vi "waitForRisEdge.vi"(3 "delay(ticks)":u32, 4 "MCSSelectTrigger":T1) -> (1 "out":bool, 2 "triggered?":bool)   [LabVIEW 2014]
uses:
  Controls/selectTrigger.ctl
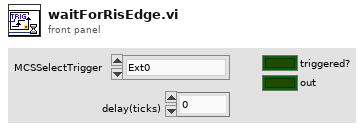
[diagram p1: front panel]
types:
  T1 = typedef "selectTrigger.ctl" = enum8{"Ext0", "Ext1", "Ext2", "Ext3", "Ext4", "Ext5", "Ext6", "Ext7", "Int0", "Int1", "Int2", "Int3", "Int4", "Int5", "Int6", "Int7"}
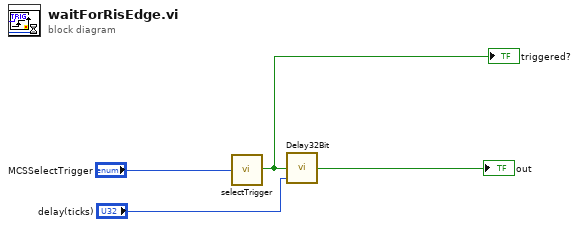
[diagram p0: block diagram]
diagram:
  n1 = call "selectTrigger.vi"("MCSSelectTrigger"="MCSSelectTrigger") -> ("risEdge"=w2:bool)  [unwired: 4 in]
  "triggered?" <- w2
  n2 = call "Delay32Bit.vi"("delay(ticks)"="delay(ticks)", "In"=w2) -> ("Out"=→"out":bool)  [unwired: 3 in]
